vi "ToString.vi"(8 "error in (no error)":errorcluster, 11 "U32 D Element in":refnum<class "Float D Element.lvclass">) -> (0 "error out":errorcluster, 2 "String":string, 3 "U32 D Element out":refnum<class "Float D Element.lvclass">)   [LabVIEW 2018, in "D Datagrid Library.lvlib" / "Float D Element.lvclass"]
uses:
  Float D Element.lvclass
  Float D Element.lvclass/Float D Element.ctl
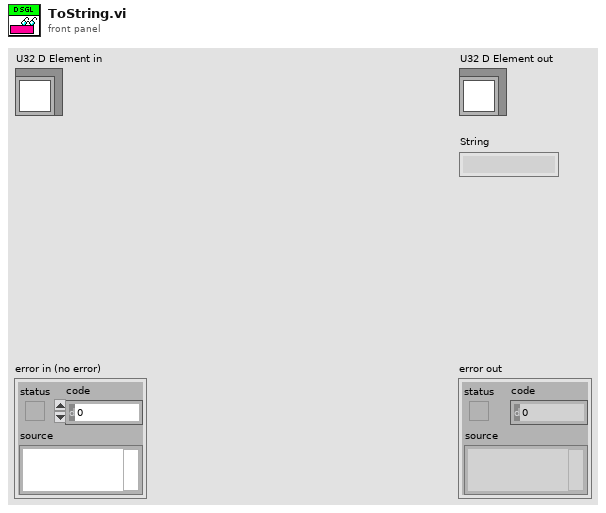
[diagram p1: front panel]
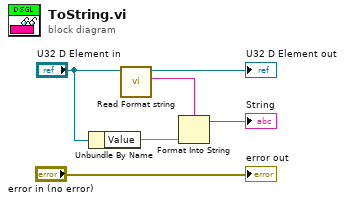
[diagram p0: block diagram]
diagram:
  n1 = Unbundle By Name("U32 D Element in") -> ("Value"=w2:sgl)
  n2 = call-dynamic "Read Format string.vi"("Float D Element in"="U32 D Element in") -> ("Format string"=w3:string, "Float D Element out"=→"U32 D Element out":refnum<class "Float D Element.lvclass">)  [unwired: 8 in, 1 out]
  n3 = Format Into String(format string=w3, w2) -> (resulting string=→"String":string)  [unwired: 2 in, 1 out]
  "error out" <- "error in (no error)"
